vi "TC Panel1 Init.vi"(10 "TC Panel 1":T1[][](array[typedef])=[[{"Label"="RDB F", "Chan"="1001", "Rec"=TRUE, "TC Label"=""}, {"Label"="Room Ambient(F)", "Chan"="1002", "Rec"=TRUE, "TC Label"=""}, {"Label"="Tscale", "Chan"="1003", "Rec"=TRUE, "TC Label"=""}, {"Label"="", "Chan"="1004", "Rec"=FALSE, "TC Label"=""}, {"Label"="", "Chan"="1005", "Rec"=FALSE, "TC Label"=""}, {"Label"="", "Chan"="1006", "Rec"=FALSE, "TC Label"=""}], [{"Label"="", "Chan"="1007", "Rec"=FALSE, "TC Label"=""}, {"Label"="", "Chan"="1008", "Rec"=FALSE, "TC Label"=""}, {"Label"="", "Chan"="1009", "Rec"=FALSE, "TC Label"=""}, {"Label"="", "Chan"="1010", "Rec"=FALSE, "TC Label"=""}, {"Label"="", "Chan"="1011", "Rec"=FALSE, "TC Label"=""}, {"Label"="", "Chan"="1012", "Rec"=FALSE, "TC Label"=""}], [{"Label"="", "Chan"="1013", "Rec"=FALSE, "TC Label"=""}, {"Label"="", "Chan"="1014", "Rec"=FALSE, "TC Label"=""}, {"Label"="", "Chan"="1015", "Rec"=FALSE, "TC Label"=""}, {"Label"="", "Chan"="1016", "Rec"=FALSE, "TC Label"=""}, {"Label"="", "Chan"="1017", "Rec"=FALSE, "TC Label"=""}, {"Label"="", "Chan"="1018", "Rec"=FALSE, "TC Label"=""}]]) -> (2 "TC Panel 1 Out":T1[][](array[typedef]))   [LabVIEW 2012]
uses:
  Dryer Performance/DPT Channel Label.ctl
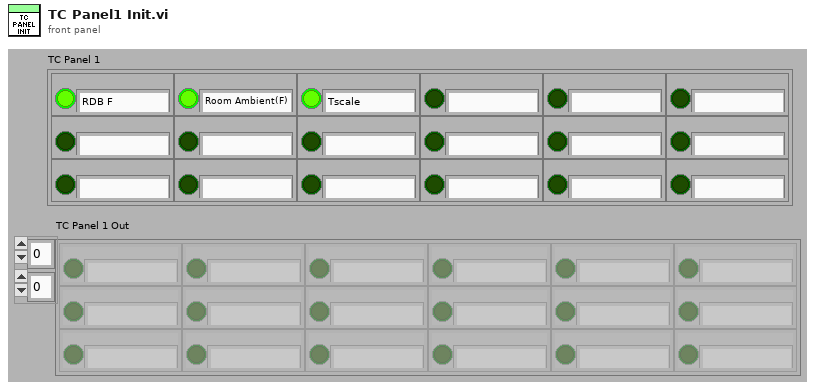
[diagram p1: front panel]
types:
  T1 = typedef "DPT Channel Label.ctl" = cluster{"Label":string, "Chan":string, "Rec":bool, "TC Label":string}
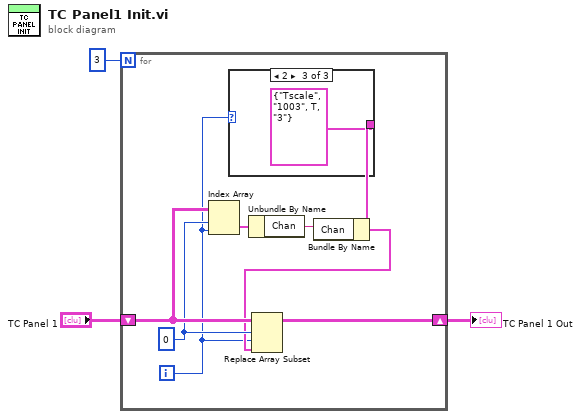
[diagram p0: block diagram]
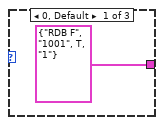
[diagram p2: hidden frame]
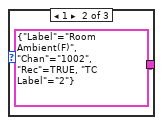
[diagram p3: hidden frame]
diagram:
  n1 = for {
    N: 3 -> [_]
    shift-right: [w11] -> w1
    shift-left: "TC Panel 1" -> [w10]
    i -> [w4]
    w9 = 0 ("index (row)")
    n2 = Index Array(array=w10, index (row)=w9, index (col)=w4) -> (element=w8:T1)
    n3 = case shown="2" w4 {
      tunnel: [T1 {"Label"="RDB F", "Chan"="1001", "Rec"=TRUE, "TC Label"="1"} ("Sensor 2") T1 {"Label"="Room Ambient(F)", "Chan"="1002", "Rec"=TRUE, "TC Label"="2"} ("Sensor 2") T1 {"Label"="Tscale", "Chan"="1003", "Rec"=TRUE, "TC Label"="3"} ("Sensor 2")] -> w5
      frame 0, Default {
      }
      frame 1 {
      }
      frame 2 {
      }
    }
    n4 = Unbundle By Name(w8) -> ("Chan"=w7:string)
    n5 = Bundle By Name(cluster=w5, "Chan"=w7) -> (w6:T1)
    n6 = Replace Array Subset(array=w10, new element=w6, index (row)=w9, index (col)=w4) -> (w11:T1[][])
  }
  "TC Panel 1 Out" <- w1
